vi "MTM2_putSample_axialEncoderPositions.vi"(8 "error in (no error)":errorcluster, 11 "axialEncoderPositions_Ctl":T1={"private_rcvStamp"=0.0, "position[72]"=[0.0, 0.0, 0.0, 0.0, 0.0, 0.0, 0.0, 0.0, 0.0, 0.0, 0.0, 0.0, 0.0, 0.0, 0.0, 0.0, 0.0, 0.0, 0.0, 0.0, 0.0, 0.0, 0.0, 0.0, 0.0, 0.0, 0.0, 0.0, 0.0, 0.0, 0.0, 0.0, 0.0, 0.0, 0.0, 0.0, 0.0, 0.0, 0.0, 0.0, 0.0, 0.0, 0.0, 0.0, 0.0, 0.0, 0.0, 0.0, 0.0, 0.0, 0.0, 0.0, 0.0, 0.0, 0.0, 0.0, 0.0, 0.0, 0.0, 0.0, 0.0, 0.0, 0.0, 0.0, 0.0, 0.0, 0.0, 0.0, 0.0, 0.0, 0.0, 0.0]}) -> (0 "error out":errorcluster, 2 "function return":i32, 3 "axialEncoderPositions_Ctl out":T1)   [LabVIEW 2018, in "SALLV_MTM2.lvlib"]
doc: "int MTM2_shm_putSample_axialEncoderPositionsLV(MTM2_axialEncoderPositionsLV *axialEncoderPositions_Ctl );"
uses:
  DataTypes/axialEncoderPositions.ctl
  SALLV_MTM2.lvlib
  SALLV_MTM2.so
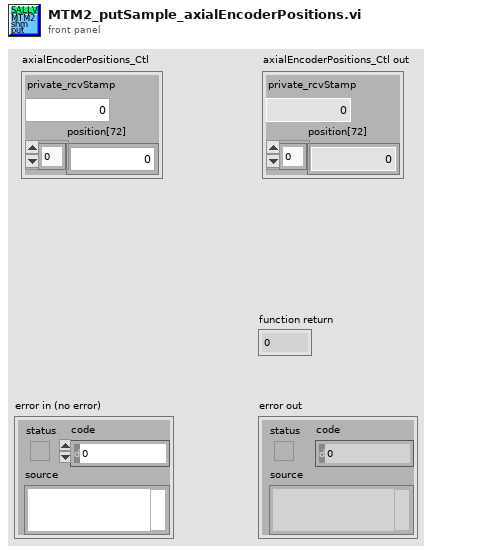
[diagram p1: front panel]
types:
  T1 = typedef "SALLV_MTM2.lvlib/axialEncoderPositions.ctl" = cluster{"private_rcvStamp":dbl, "position[72]":dbl[]}
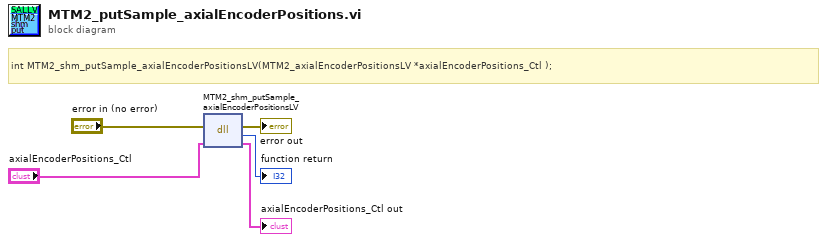
[diagram p0: block diagram]
diagram:
  # "int MTM2_shm_putSample_axialEncoderPositionsLV(MTM2_axialEncoderPositionsLV *axialEncoderPositions_Ctl );"
  n1 = dll-call lib="home/ttsai/Documents/salTestLabViewApi/SALLV_MTM2/SALLV_MTM2.*" fn="MTM2_shm_putSample_axialEncoderPositionsLV"(error in="error in (no error)", "axialEncoderPositions_Ctl"="axialEncoderPositions_Ctl") -> (error out=→"error out":errorcluster, →"function return":i32, "axialEncoderPositions_Ctl"=→"axialEncoderPositions_Ctl out":T1)  [unwired: 2 in, 1 out]
